vi "Scaled Random Number.vi"(10 "Low":i32, 11 "High":i32=1) -> (3 "Scaled Random Number":dbl)   [LabVIEW 2011]
doc: "Generates a scaled random number.\n\n\nVersion 1.0 - 10/21/2009\n\nPhaeron, Inc.\nwww.phaeron.com\ninfo@phaeron.com"
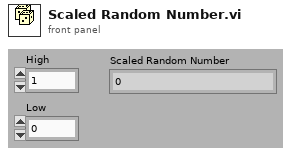
[diagram p1: front panel]
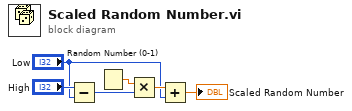
[diagram p0: block diagram]
diagram:
  n1 = Subtract(x="High", y="Low") -> (x-y=w5:i32)
  n2 = Random Number (0-1)() -> (number: 0 to 1=w4:dbl)
  n3 = Multiply(x=w4, y=w5) -> (x*y=w3:dbl)
  n4 = Add(x=w3, y="Low") -> (x+y=→"Scaled Random Number":dbl)
